vi "ExecuteSkill.vi"(0 "object in":refnum<class "PassSkill.lvclass">, 2 "Robot in":refnum<class "Robot.lvclass">, 4 "GameRef":refnum<data-value>, 5 "error in (no error)":errorcluster) -> (14 "object out":refnum<class "PassSkill.lvclass">, 16 "Robot out":refnum<class "Robot.lvclass">, 19 "error out":errorcluster)   [LabVIEW 2023, in "PassSkill.lvclass"]
uses:
  PassSkill.lvclass
  C:/Users/ebert/Documents/codes/SSL/repo/SSL_AI/KickToSkill_v2_class/KickToSkill_v2.lvclass
  Robot_class/Robot.lvclass
  Game_class/Game.lvclass
  KickToSkill_v2_class/KickToSkill_v2.lvclass
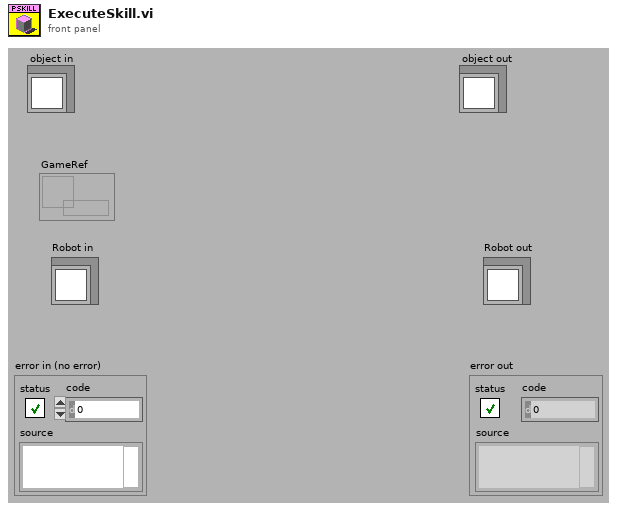
[diagram p1: front panel]
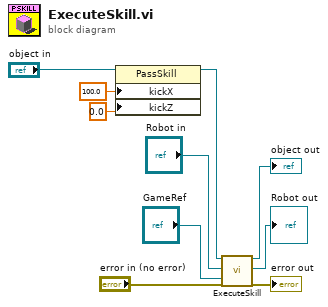
[diagram p0: block diagram]
diagram:
  n1 = property class="PassSkill"(reference="object in", "kickX"=100.0, "kickZ"=0.0) -> (reference out=w3:refnum<class "PassSkill.lvclass">)  [unwired: 1 in, 1 out]
  n2 = call-parent "ExecuteSkill.vi"("object in"=w3, "Robot in"="Robot in", "GameRef"="GameRef", "error in (no error)"="error in (no error)") -> ("object out"=→"object out":refnum<class "PassSkill.lvclass">, "Robot out"=→"Robot out":refnum<class "Robot.lvclass">, "error out"=→"error out":errorcluster)  [unwired: 13 in]
